vi "NumberChanger.vi"(0 "Input":u64) -> (1 "New Value":u64, 2 "Value 2":u64)   [LabVIEW 2014]
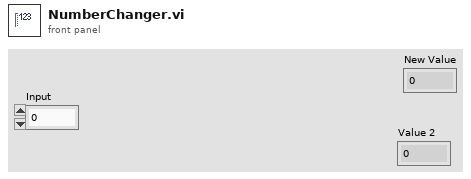
[diagram p1: front panel]
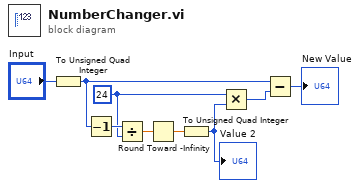
[diagram p0: block diagram]
diagram:
  w3 = u64 24 ("y")
  n1 = To Unsigned Quad Integer(1:"Input") -> (0:w2:u64)
  n2 = Decrement(x=w2) -> (x-1=w8:u64)
  n3 = Divide(x=w8, y=w3) -> (x/y=w7:dbl)
  n4 = Round Toward -Infinity(1:w7) -> (0:w6:dbl)
  n5 = To Unsigned Quad Integer(1:w6) -> (0:w4:u64)
  "Value 2" <- w4
  n6 = Multiply(x=w3, y=w4) -> (x*y=w5:u64)
  n7 = Subtract(x=w2, y=w5) -> (x-y=→"New Value":u64)
